vi "Queued Frame to Normal Frame.vi"(10 "CAN frame in":T2 {"type" items=["CAN Data", "CAN Remote"]}) -> (2 "CAN frame out":T1 {"type" items=["CAN Data", "CAN Remote"]; "identifier" format="%.0x"})   [LabVIEW 2014]
uses:
  CAN Message.ctl
  <vilib>/RioEmbeddedCAN/RioEmbeddedCAN.llb/CANFrameControl.ctl
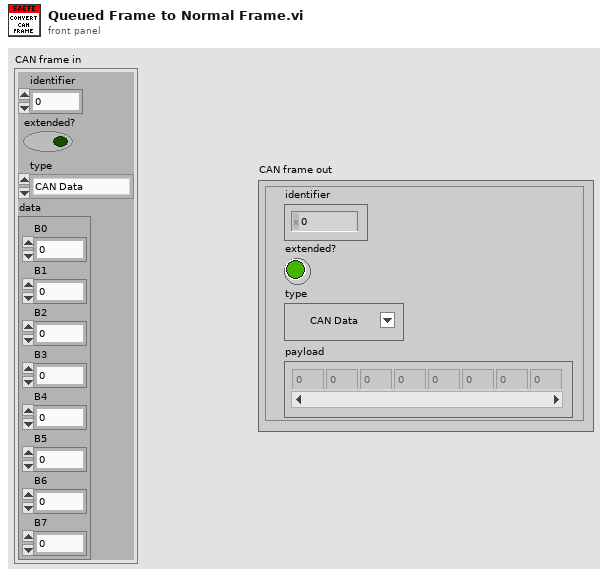
[diagram p1: front panel]
types:
  T1 = typedef "CANFrameControl.ctl" = cluster{"identifier":u32, "extended?":bool, "type":u8, "payload":u8[]}
  T2 = typedef "CAN Message.ctl" = cluster{"identifier":u32, "extended?":bool, "type":u8, "data":cluster{"B0":u8, "B1":u8, "B2":u8, "B3":u8, "B4":u8, "B5":u8, "B6":u8, "B7":u8}}
  T3 = cluster{"identifier":u32, "extended?":bool, "type":u8, "payload":u8[]}
  T4 = cluster{"B0":u8, "B1":u8, "B2":u8, "B3":u8, "B4":u8, "B5":u8, "B6":u8, "B7":u8}
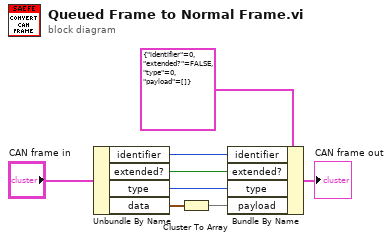
[diagram p0: block diagram]
diagram:
  n1 = Unbundle By Name("CAN frame in") -> ("identifier"=w5:u32, "extended?"=w4:bool, "type"=w3:u8, "data"=w2:T4)
  n2 = Cluster To Array(cluster=w2) -> (array=w1:u8[])
  n3 = Bundle By Name(cluster=T3 {"identifier"=0, "extended?"=FALSE, "type"=0, "payload"=[]} ("CAN frame"), "identifier"=w5, "extended?"=w4, "type"=w3, "payload"=w1) -> (→"CAN frame out":T3)
